vi "SetDUTport.vi"(6 "Legacy (f)?":bool, 8 "error in (no error)":errorcluster, 10 "SetDUTport":T1) -> (0 "error out":errorcluster)   [LabVIEW 2011]
uses:
  DUTport.ctl
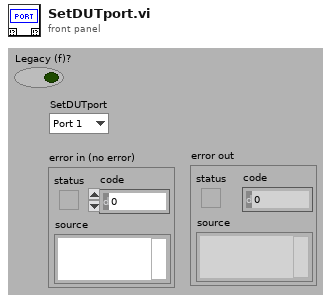
[diagram p1: front panel]
types:
  T1 = typedef "DUTport.ctl" = enum16{"Port 1", "Port 2"}
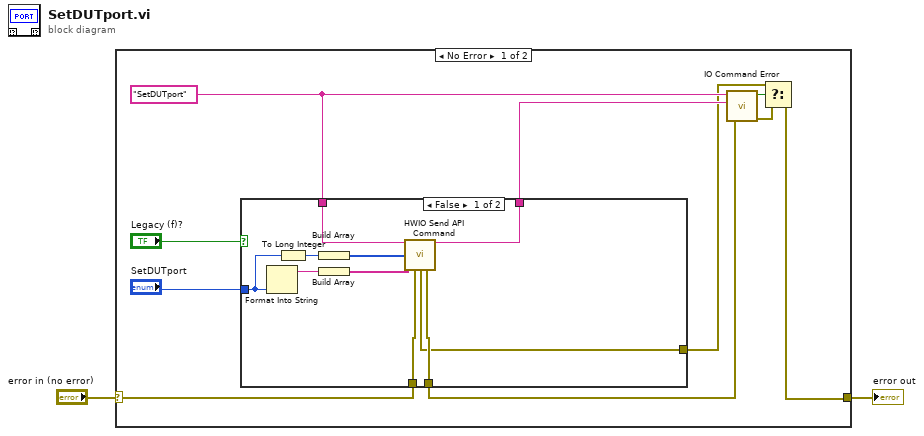
[diagram p0: block diagram]
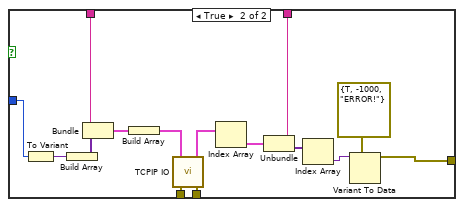
[diagram p2: hidden frame]
diagram:
  n1 = case shown="No Error" "error in (no error)" {
    selector: "error in (no error)" -> [w8 w38]
    tunnel: [w5 w38] -> w2
    frame No Error {
      w10 = "SetDUTport"
      n2 = case shown="False" "Legacy (f)?" {
        tunnel: "SetDUTport" -> [w18 w35]
        tunnel: [w20 w32] -> w11
        tunnel: w10 -> [w21 w31]
        tunnel: [w14 w30] -> w9
        tunnel: w8 -> [w22 w27]
        tunnel: [w13 w24] -> w3
        frame False {
          n3 = Format Into String(w18) -> (resulting string=w17:string)  [unwired: 3 in, 1 out]
          n4 = To Long Integer(number=w18) -> (32bit integer=w19:i32)
          n5 = Build Array(w19) -> (w16:i32[])
          n6 = Build Array(w17) -> (w15:string[])
          n7 = call "HWIO Send API Command.vi"("Action"=w21, "Integer"=w16, "String"=w15, "error in (no error)"=w22) -> ("Action out"=w20:string, "HWError"=w13:errorcluster, "error out"=w14:errorcluster)  [unwired: 4 in, 5 out]
        }
        frame True {
          n8 = To Variant(anything=w35) -> (Variant=w37:variant)
          n9 = Build Array(w37) -> (w36:variant[])
          n10 = Bundle(w31, w36) -> (w33:cluster{string, variant[]})  [unwired: 1 out]
          n11 = Build Array(w33) -> (w34:cluster{string, variant[]}[])
          n12 = call "TCPIP IO.vi"("error in (no error)"=w27, "Commands"=w34) -> ("error out"=w30:errorcluster, "Responses"=w28:cluster{string, variant[]}[])  [unwired: 1 in, 3 out]
          n13 = Index Array(array=w28) -> (element=w29:cluster{string, variant[]})  [unwired: 1 in]
          n14 = Unbundle(w29) -> (w32:string, w23:variant[])
          n15 = Index Array(array=w23) -> (element=w26:variant)  [unwired: 1 in]
          n16 = Variant To Data(type=errorcluster {"status"=TRUE, "code"=-1000, "source"="ERROR!"} ("error out"), Variant=w26) -> (data=w24:errorcluster)  [unwired: 1 in, 1 out]
        }
      }
      n17 = call "IO Command Error.vi"("error in (no error)"=w9, "Command Returned (\"\")"=w11, "Command Sent (\"\")"=w10) -> ("error out"=w6:errorcluster, "HW ERR?"=w7:bool)  [unwired: 3 out]
      n18 = Select(t=w3, s=w7, f=w6) -> (s? t:f=w5:errorcluster)
    }
    frame Error {
    }
  }
  "error out" <- w2
